vi "RotationAlignment.vi"(10 "Right Distance":dbl, 11 "Left Distance":dbl) -> (2 "Right Motor":dbl, 3 "Left Motor":dbl)   [LabVIEW 2018]
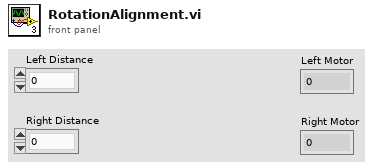
[diagram p1: front panel]
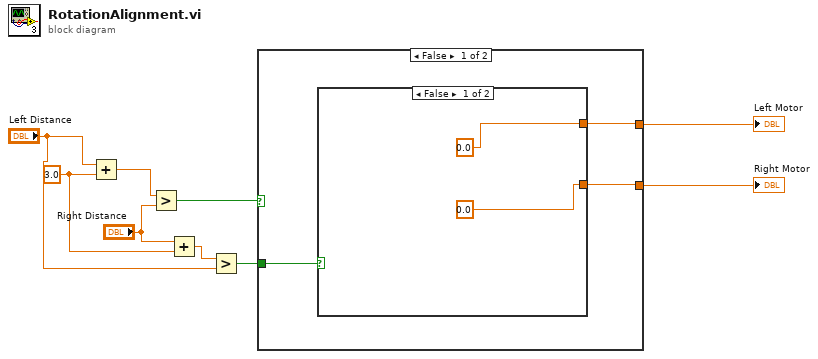
[diagram p0: block diagram]
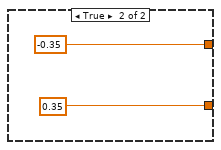
[diagram p2: hidden frame]
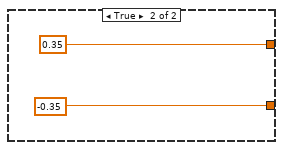
[diagram p3: hidden frame]
diagram:
  w5 = 3.0 ("y")
  n1 = Add(x="Left Distance", y=w5) -> (x+y=w9:dbl)
  n2 = Greater?(x=w9, y="Right Distance") -> (0:w8:bool)
  n3 = Add(x="Right Distance", y=w5) -> (x+y=w2:dbl)
  n4 = Greater?(x=w2, y="Left Distance") -> (0:w1:bool)
  n5 = case shown="False" w8 {
    tunnel: [w10 0.35 ("Left Motor")] -> w7
    tunnel: [w11 -0.35 ("Left Motor")] -> w6
    tunnel: w1 -> [w12 _]
    frame False {
      n6 = case shown="False" w12 {
        tunnel: [0.0 ("Left Motor") -0.35 ("Left Motor")] -> w10
        tunnel: [0.0 ("Left Motor") 0.35 ("Left Motor")] -> w11
        frame False {
        }
        frame True {
        }
      }
    }
    frame True {
    }
  }
  "Left Motor" <- w7
  "Right Motor" <- w6
